vi "Validation App.vi"() -> ()   [LabVIEW 2020, in "VolatusConfig.lvlib"]
uses:
  VolatusConfig.lvlib
  VolatusConfig/VolatusConfig.lvclass
panel:
  out "File":string
  in  "Revalidate":bool
  in  "Load":bool
  out "Message":string
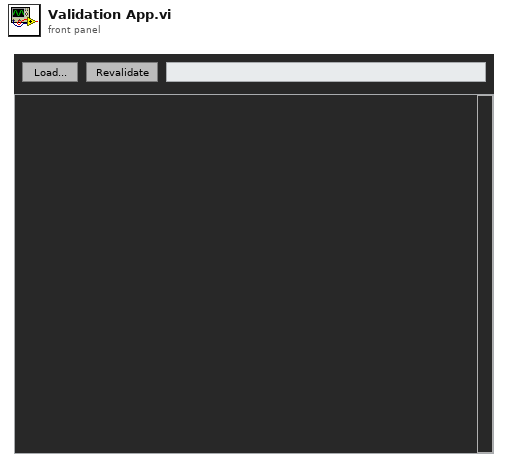
[diagram p1: front panel]
types:
  T1 = typedef "VolatusConfig.lvlib/Config Format.ctl" = enum16{"JSON", "INI", "SQLite"}
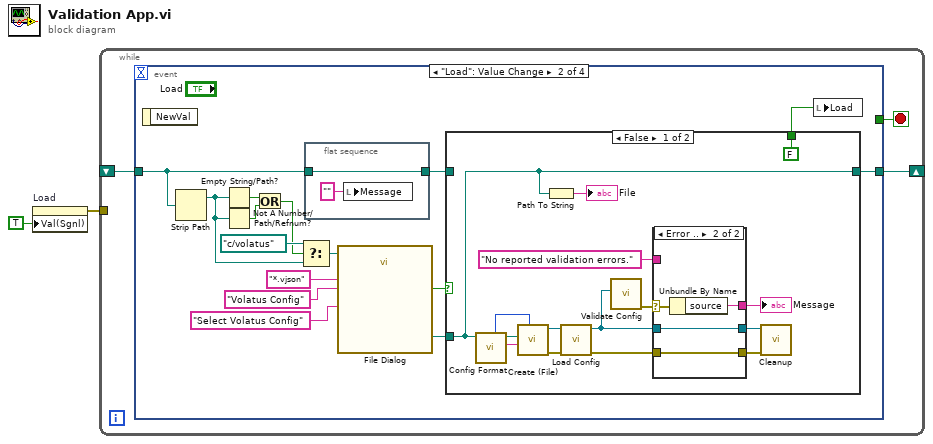
[diagram p0: block diagram]
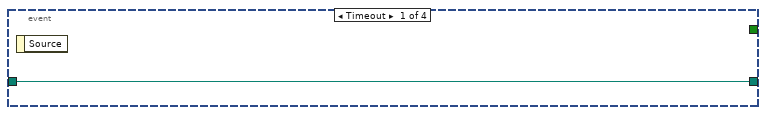
[diagram p2: hidden frame]
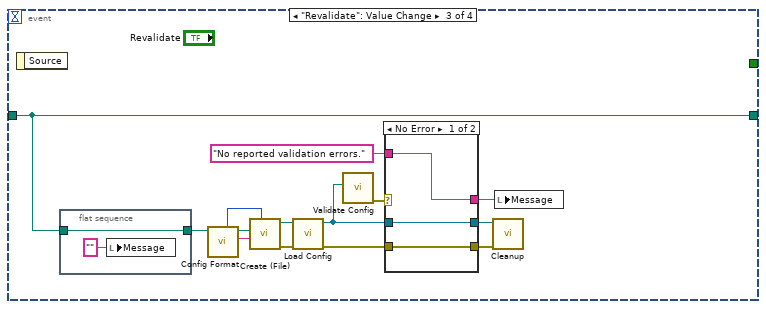
[diagram p5: hidden frame]
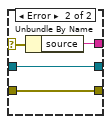
[diagram p6: hidden frame]
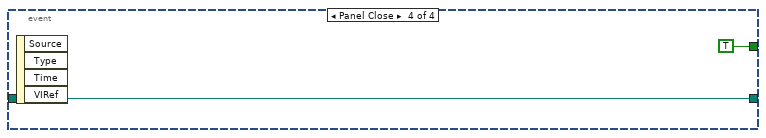
[diagram p7: hidden frame]
diagram:
  n1 = property on="Load" class="Bool (strict)"("Val(Sgnl)"=TRUE ("Value (Signaling)")) -> (error out=w2:errorcluster)  [unwired: 2 in, 1 out]
  n2 = while {
    shift-right: [w4] -> _
    shift-left: _ -> [w3]
    tunnel: w2 -> [_]
    stop <- w5 stop-if-true
    n3 = event shown="[1] \"Load\": Value Change" {
      selector: _ -> [_ _ _ _]
      dyn-events: _ -> [_ _ _ _]
      timeout: _ -> [_ _ _ _]
      tunnel: [_ _ _ TRUE] -> w5
      tunnel: [w6 w10 w47 w70] -> w4
      tunnel: w3 -> [w6 w8 w47 w70]
      event Timeout {
        n4 = event-data() -> ()  [unwired: 1 in, 1 out]
      }
      event "Load": Value Change {
        n5 = event-data() -> ()  [unwired: 1 in, 1 out]
        n6 = Strip Path(path=w8) -> (stripped path=w13:path)  [unwired: 1 out]
        n7 = Empty String/Path?(string/path=w13) -> (empty?=w17:bool)
        n8 = Not A Number/Path/Refnum?(number/path/refnum=w13) -> (NaN/Path/Refnum?=w16:bool)
        n9 = Or(x=w17, y=w16) -> (x .or. y?=w15:bool)
        n10 = Select(t=path "c:/volatus", s=w15, f=w13) -> (s? t:f=w14:path)
        n11 = flat-sequence {
          tunnel: [w22] -> w9
          tunnel: w8 -> [w22]
          frame #0 {
            n12 = local write "Message"("" ("Message")) -> ()
          }
        }
        n13 = call "File Dialog"("start path"=w14, "prompt"="Select Volatus Config", "pattern (all files)"="*.vjson", "pattern label"="Volatus Config") -> ("selected path"=w12:path, "cancelled"=w11:bool)  [unwired: 8 in, 2 out]
        n14 = case shown="False" w11 {
          tunnel: w12 -> [w26 _]
          tunnel: w9 -> [_ w46]
          tunnel: [w26 w46] -> w10
          tunnel: [FALSE _] -> w7
          frame False {
            n15 = call "Config Format.vi"("Config Path"=w26) -> ("filename without extension"=w36:string, "Folder"=w37:path, "Format"=w38:T1)  [unwired: 8 in]
            n16 = call "Create (File).vi"("Main Format"=w38, "Main Filename"=w36, "Config Root"=w37) -> ("error out"=w34:errorcluster, "VolatusConfig out"=w35:refnum<class "VolatusConfig.lvclass">)  [unwired: 7 in]
            n17 = Path To String(path=w26) -> (string=→"File":string)
            n18 = call "Load Config.vi"("error in (no error)"=w34, "VolatusConfig in"=w35) -> ("error out"=w33:errorcluster, "VolatusConfig out"=w29:refnum<class "VolatusConfig.lvclass">)  [unwired: 7 in, 1 out]
            n19 = call "Validate Config.vi"("VolatusConfig"=w29) -> ("error out"=w32:errorcluster)  [unwired: 10 in]
            n20 = case shown="Error .." w32 {
              selector: w32 -> [_ w43]
              tunnel: w33 -> [w41 w44]
              tunnel: [w41 w44] -> w31
              tunnel: [w40 w45] -> w30
              tunnel: w29 -> [w40 w45]
              tunnel: [w39 w42] -> w28
              tunnel: "No reported validation errors." -> [w39 _]
              frame No Error {
              }
              frame Error {
                n21 = Unbundle By Name(w43) -> ("source"=w42:string)
              }
            }
            "Message" <- w28
            n22 = call "Cleanup.vi"("error in (no error)"=w31, "VolatusConfig in"=w30) -> ()  [unwired: 9 in, 1 out]
          }
          frame True {
          }
        }
        n23 = local write "Load"(w7) -> ()
      }
      event "Revalidate": Value Change {
        n24 = event-data() -> ()  [unwired: 1 in, 1 out]
        n25 = flat-sequence {
          tunnel: [w61] -> w48
          tunnel: w47 -> [w61]
          frame #0 {
            n26 = local write "Message"("" ("Message")) -> ()
          }
        }
        n27 = call "Config Format.vi"("Config Path"=w48) -> ("filename without extension"=w58:string, "Folder"=w59:path, "Format"=w60:T1)  [unwired: 8 in]
        n28 = call "Create (File).vi"("Main Format"=w60, "Main Filename"=w58, "Config Root"=w59) -> ("error out"=w56:errorcluster, "VolatusConfig out"=w57:refnum<class "VolatusConfig.lvclass">)  [unwired: 7 in]
        n29 = call "Load Config.vi"("error in (no error)"=w56, "VolatusConfig in"=w57) -> ("error out"=w55:errorcluster, "VolatusConfig out"=w51:refnum<class "VolatusConfig.lvclass">)  [unwired: 7 in, 1 out]
        n30 = call "Validate Config.vi"("VolatusConfig"=w51) -> ("error out"=w54:errorcluster)  [unwired: 10 in]
        n31 = case shown="No Error" w54 {
          selector: w54 -> [_ w67]
          tunnel: w55 -> [w65 w68]
          tunnel: [w65 w68] -> w53
          tunnel: [w64 w69] -> w52
          tunnel: w51 -> [w64 w69]
          tunnel: [w63 w66] -> w49
          tunnel: "No reported validation errors." -> [w63 _]
          frame No Error {
          }
          frame Error {
            n32 = Unbundle By Name(w67) -> ("source"=w66:string)
          }
        }
        n33 = call "Cleanup.vi"("error in (no error)"=w53, "VolatusConfig in"=w52) -> ()  [unwired: 9 in, 1 out]
        n34 = local write "Message"(w49) -> ()
      }
      event Panel Close {
        n35 = event-data() -> ()  [unwired: 1 in, 4 out]
      }
    }
  }
